vi "Stop.vi"(8 "error in (no error)":errorcluster, 11 "Topic Actor Command Interface in":refnum<class "Topic Actor Command Interface.lvclass">) -> (0 "error out":errorcluster, 2 "Stop?":bool, 3 "Topic Actor Command Interface out":refnum<class "Topic Actor Command Interface.lvclass">)   [LabVIEW 2016, in "Stream Mediator.lvlib" / "Topic Actor Command Interface.lvclass"]
doc: "--\nCopyright © 2017 Composed SystemsI All rights reserved.\n\nAuthor: Jon McBee <jon.mcbee@composed.io>\n\nThis library is provided \"AS IS\" ,WITHOUT WARRANTIES OR\nCONDITIONS OF ANY KIND, either express or implied.\n\nComposed Systems -- composed.io\n\nStream 0.0.1.1\nJon McBee - Composed Systems\nCopyright (c) 2017, Composed Systems"
uses:
  <userlib>/Composed Systems/Stream/Mediator/Classes/Topic Actor Command Interface/Topic Actor Command Interface.lvclass
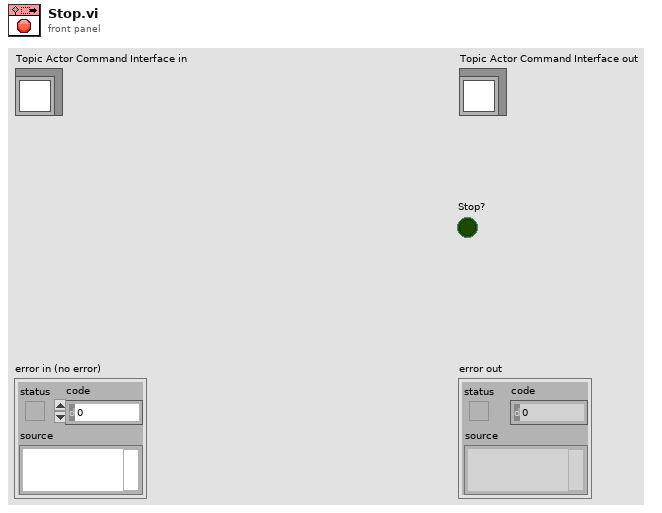
[diagram p1: front panel]
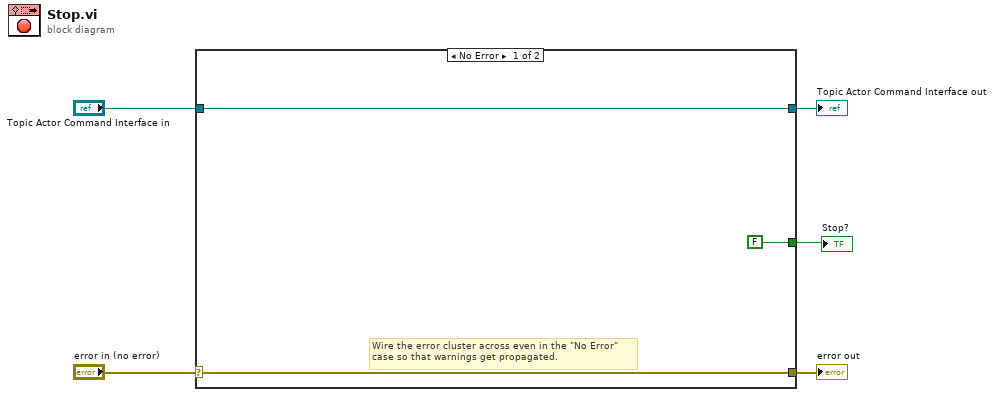
[diagram p0: block diagram]
diagram:
  n1 = case shown="No Error" "error in (no error)" {
    selector: "error in (no error)" -> [w7 w10]
    tunnel: [w7 w10] -> w4
    tunnel: [w8 w9] -> w2
    tunnel: "Topic Actor Command Interface in" -> [w8 w9]
    tunnel: [FALSE _] -> w1
    frame No Error {
      # "Wire the error cluster across even in the \"No Error\"\ncase so that warnings get propagated."
    }
    frame Error {
    }
  }
  "error out" <- w4
  "Topic Actor Command Interface out" <- w2
  "Stop?" <- w1
